vi "Deserialise content.vi"(8 "error in (no error)":errorcluster, 10 "JSON String to decode":string, 11 "object in":refnum<class "kernel_info_reply Message.lvclass">) -> (0 "error out":errorcluster, 3 "object out":refnum<class "kernel_info_reply Message.lvclass">)   [LabVIEW 2018, in "ClientMessaging.lvlib" / "kernel_info_reply Message.lvclass"]
uses:
  kernel_info_reply Message.lvclass
  kernel_info_reply Message.lvclass/kernel_info_reply Message.ctl
  2aeaedef-f14a-48fc-a4e7-757a2cfbc284.vi
  34bd3cb7-fd0b-4a33-bb86-ed73d2d1add7.vi
  2aeaedef-f14a-48fc-a4e7-757a2cfbc284.vi/966cd031-8f94-4fe2-ab59-99c1fa1a9b7e.vi
  2aeaedef-f14a-48fc-a4e7-757a2cfbc284.vi/274a14cb-3ec5-4030-a81d-321e4cab5c5e.vi
  2aeaedef-f14a-48fc-a4e7-757a2cfbc284.vi/9cc802bf-3bbd-4a23-9d7b-d56cecca5d4b.vi
  34bd3cb7-fd0b-4a33-bb86-ed73d2d1add7.vi/4761e8c6-d3e9-44ce-be32-523bf575d766.vi
  34bd3cb7-fd0b-4a33-bb86-ed73d2d1add7.vi/3659f788-c207-4f36-8cad-c06de4114500.vi
  34bd3cb7-fd0b-4a33-bb86-ed73d2d1add7.vi/b851aadb-6241-46a9-90b8-486c78f15aae.vi
  <vilib>/JDP Science/JSONtext/Find Item.vi
  <vilib>/JDP Science/JSONtext/String Subset.vi
  <vilib>/JDP Science/JSONtext/Parsing/Parse Full Path or Item Name.vi
  <vilib>/JDP Science/JSONtext/Offset/Find Item Locations by Path.vi
  <vilib>/JDP Science/JSONtext/JSON text to Variant.vi
  Utility/Join Strings in node-path.vi
  Base Classes/Reply Message/Reply Message.lvclass
  Base Classes/Message Class/Message Class.lvclass
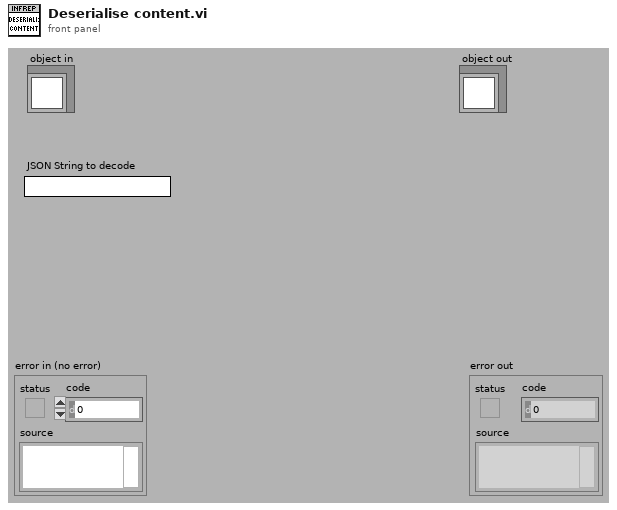
[diagram p1: front panel]
types:
  T1 = cluster{"[0]":string, "[1]":string, "[2]":string, "[3]":string, "[4]":string, "[5]":string, "[6]":string}
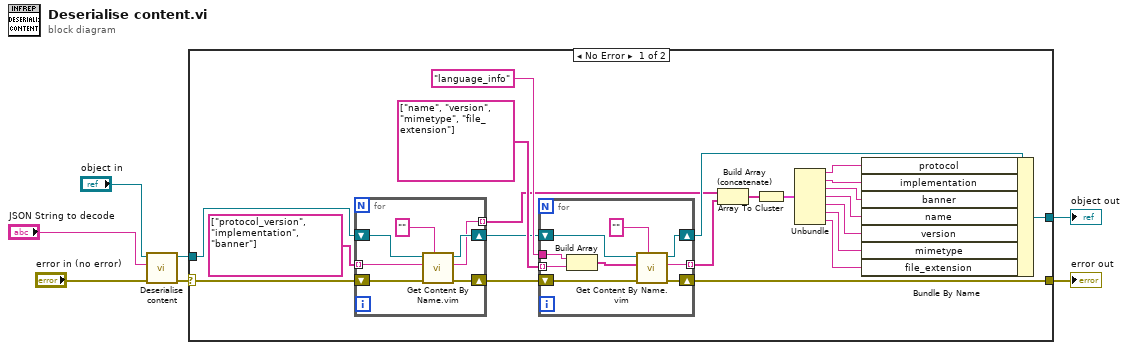
[diagram p0: block diagram]
diagram:
  n1 = call-parent "Deserialise content.vi"("error in (no error)"="error in (no error)", "JSON String to decode"="JSON String to decode", "object in"="object in") -> ("error out"=w1:errorcluster, "object out"=w4:refnum<class "kernel_info_reply Message.lvclass">)  [unwired: 7 in]
  n2 = case shown="No Error" w1 {
    selector: w1 -> [w23 w46]
    tunnel: [w19 w46] -> w7
    tunnel: [w27 w45] -> w5
    tunnel: w4 -> [w28 w45]
    frame No Error {
      n3 = for {
        tunnel: string[] ["protocol_version", "implementation", "banner"] -> [w43] mode=indexing
        shift-right: [w40] -> w22
        shift-left: w28 -> [w44]
        shift-right: [w39] -> w21
        shift-left: w23 -> [w41]
        tunnel: [w38] -> w18 mode=indexing
        n4 = call "Get Content By Name.vim"("Type of content"="", "error in (no error)"=w41, "Name of Content Item"=w43, "Message In"=w44) -> ("error out"=w39:errorcluster, "Data Out"=w38:string, "Message Out"=w40:refnum<class "kernel_info_reply Message.lvclass">)  [unwired: 5 in]
      }
      n5 = for {
        tunnel: "language_info" -> [w37]
        tunnel: string[] ["name", "version", "mimetype", "file_extension"] -> [w36] mode=indexing
        shift-right: [w31] -> w20
        shift-left: w22 -> [w34]
        shift-right: [w30] -> w19
        shift-left: w21 -> [w32]
        tunnel: [w29] -> w17 mode=indexing
        n6 = Build Array(w37, w36) -> (w35:string[])
        n7 = call "Get Content By Name.vim"("Type of content"="", "error in (no error)"=w32, "Name of Content Item"=w35, "Message In"=w34) -> ("error out"=w30:errorcluster, "Data Out"=w29:string, "Message Out"=w31:refnum<class "kernel_info_reply Message.lvclass">)  [unwired: 5 in]
      }
      n8 = Build Array (concatenate)(w18, w17) -> (w16:string[])
      n9 = Array To Cluster(array=w16) -> (cluster=w15:T1)
      n10 = Unbundle(w15) -> ("[0]"=w14:string, "[1]"=w13:string, "[2]"=w12:string, "[3]"=w11:string, "[4]"=w10:string, "[5]"=w9:string, "[6]"=w8:string)
      n11 = Bundle By Name(cluster=w20, "protocol"=w14, "implementation"=w13, "banner"=w12, "name"=w11, "version"=w10, "mimetype"=w9, "file_extension"=w8) -> (w27:refnum<class "kernel_info_reply Message.lvclass">)
    }
    frame Error {
    }
  }
  "error out" <- w7
  "object out" <- w5
